vi "Pack Message.vi"(8 "error in (no error)":errorcluster, 11 "Data Message Interface in":refnum<class "Data Message Interface.lvclass">) -> (0 "error out":errorcluster, 1 "Packed Message":string, 2 "Message Name":string, 3 "Data Message Interface out":refnum<class "Data Message Interface.lvclass">)   [LabVIEW 2016, in "Stream Mediator.lvlib" / "Data Message Interface.lvclass"]
uses:
  <userlib>/Composed Systems/Stream/Mediator/Classes/Message Data Interface/Data Message Interface.lvclass
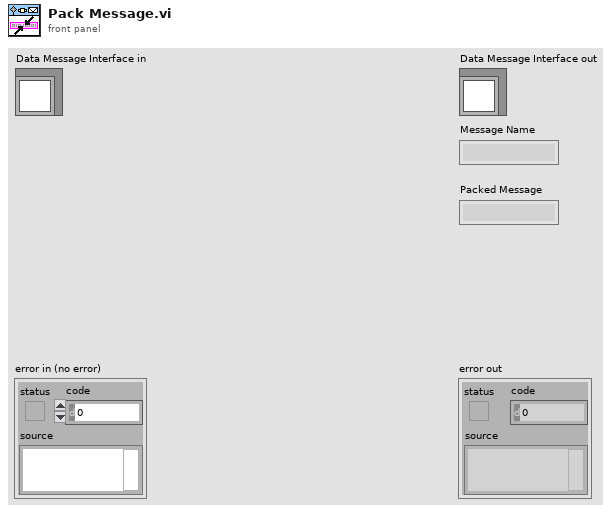
[diagram p1: front panel]
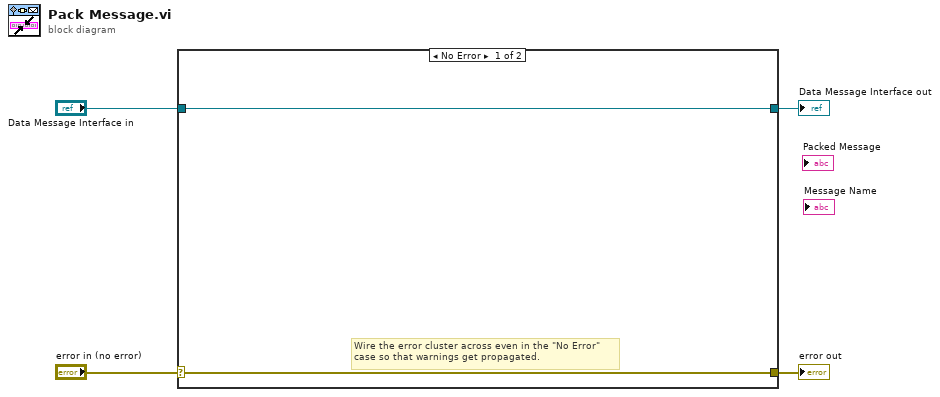
[diagram p0: block diagram]
diagram:
  n1 = case shown="No Error" "error in (no error)" {
    selector: "error in (no error)" -> [w5 w8]
    tunnel: [w5 w8] -> w3
    tunnel: [w6 w7] -> w1
    tunnel: "Data Message Interface in" -> [w6 w7]
    frame No Error {
      # "Wire the error cluster across even in the \"No Error\"\ncase so that warnings get propagated."
    }
    frame Error {
    }
  }
  "error out" <- w3
  "Data Message Interface out" <- w1
